vi "storeArgVarAndSecVarForEachRow.vi"(10 "allArguments":string="Bel_LTM_Auto,*value_Bel_LTM_Auto,1", 11 "func":string="signalSetting") -> (2 "secVar":string[](array[string]), 3 "argVar":string[](array[string])=["value_Bel_LTM_Auto"])   [LabVIEW 2010]
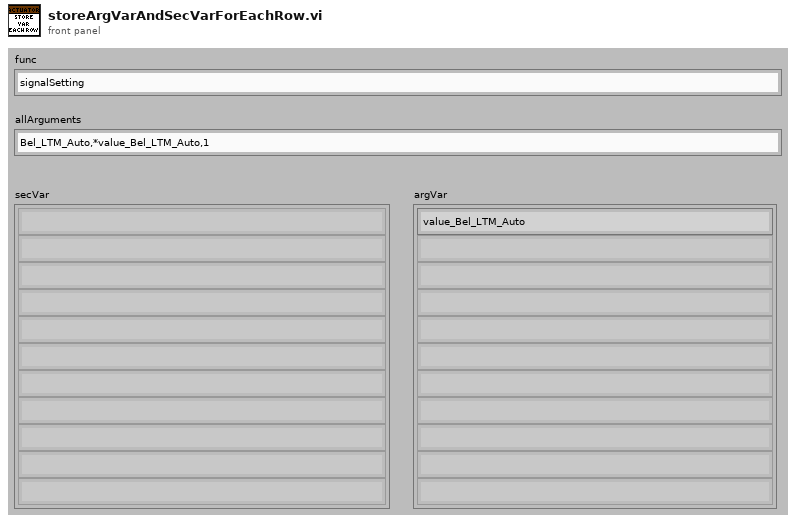
[diagram p1: front panel]
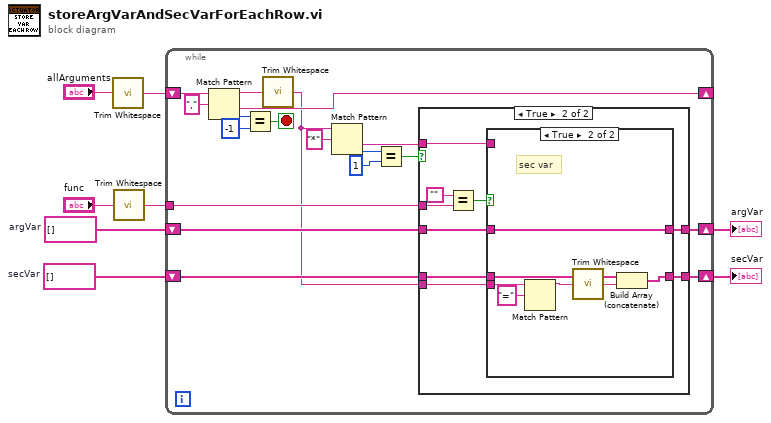
[diagram p0: block diagram]
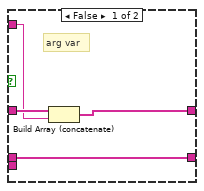
[diagram p3: hidden frame]
diagram:
  w3 = string[] []  # secVar
  w6 = string[] []  # argVar
  n1 = call <vilib>:"Trim Whitespace.vi"("string"="allArguments") -> ("trimmed string"=w7:string)  [unwired: 1 in]
  n2 = call <vilib>:"Trim Whitespace.vi"("string"="func") -> ("trimmed string"=w4:string)  [unwired: 1 in]
  n3 = while {
    shift-right: [w22] -> _
    shift-left: w7 -> [w26]
    shift-right: [w12] -> w1
    shift-left: w6 -> [w17]
    tunnel: w4 -> [w18]
    shift-right: [w9] -> w2
    shift-left: w3 -> [w11]
    stop <- w21 stop-if-true
    n4 = Match Pattern(string=w26, regular expression=",") -> (before substring=w20:string, after substring=w22:string, offset past match=w24:i32)  [unwired: 1 in, 1 out]
    n5 = Equal?(x=w24, y=-1) -> (x = y?=w21:bool)
    n6 = call <vilib>:"Trim Whitespace.vi"("string"=w20) -> ("trimmed string"=w10:string)  [unwired: 1 in]
    n7 = Match Pattern(string=w10, regular expression="*") -> (after substring=w13:string, offset past match=w15:i32)  [unwired: 1 in, 2 out]
    n8 = Equal?(x=w15, y=1 ("length (rest)")) -> (x = y?=w19:bool)
    n9 = case shown="True" w19 {
      tunnel: w18 -> [_ w37]
      tunnel: w17 -> [w28 w34]
      tunnel: w13 -> [_ w33]
      tunnel: [w28 w32] -> w12
      tunnel: w11 -> [w27 w31]
      tunnel: w10 -> [_ w30]
      tunnel: [w27 w29] -> w9
      frame False {
        # "normal arg"
      }
      frame True {
        n10 = Equal?(x="", y=w37) -> (x = y?=w35:bool)
        n11 = case shown="True" w35 {
          tunnel: w34 -> [w41 w48]
          tunnel: w33 -> [w40 _]
          tunnel: [w39 w48] -> w32
          tunnel: w31 -> [w38 w47]
          tunnel: w30 -> [_ w45]
          tunnel: [w38 w46] -> w29
          frame False {
            # "arg var"
            n12 = Build Array (concatenate)(w41, w40) -> (w39:string[])
          }
          frame True {
            # "sec var"
            n13 = Match Pattern(string=w45, regular expression="=") -> (before substring=w43:string)  [unwired: 1 in, 3 out]
            n14 = call <vilib>:"Trim Whitespace.vi"("string"=w43) -> ("trimmed string"=w42:string)  [unwired: 1 in]
            n15 = Build Array (concatenate)(w47, w42) -> (w46:string[])
          }
        }
      }
    }
  }
  "secVar" <- w2
  "argVar" <- w1
